vi "Find and trigger default events.vi"(9 "Event to Trigger":string, 10 "Module Lib":refnum<vi>, 11 "References Map":map{string, refnum<vi>}(c390)) -> (0 "error out":errorcluster)   [LabVIEW 2020, in "Panter Dashboard.lvlib"]
uses:
  Panter Dashboard.lvlib
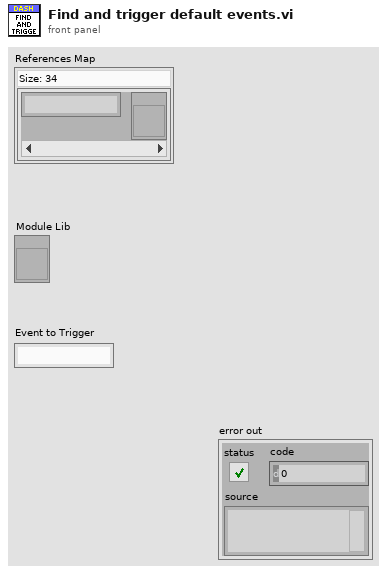
[diagram p1: front panel]
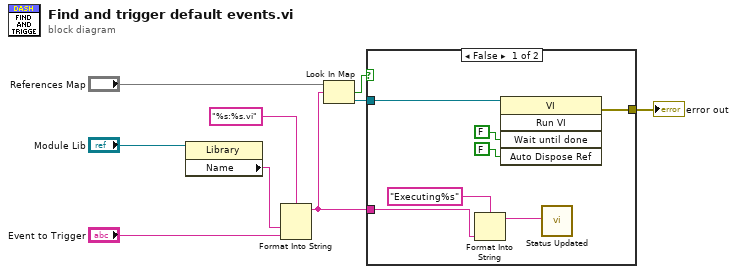
[diagram p0: block diagram]
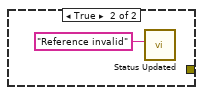
[diagram p2: hidden frame]
diagram:
  n1 = property class="Library"(reference="Module Lib") -> ("Name"=w3:string)  [unwired: 1 in, 2 out]
  n2 = Format Into String(format string="%s:%s.vi", w3, "Event to Trigger") -> (resulting string=w1:string)  [unwired: 2 in, 1 out]
  n3 = Look In Map(map="References Map", key=w1) -> (key not found?=w2:bool, value=w8:refnum<vi>)  [unwired: 1 in]
  n4 = case shown="False" w2 {
    tunnel: w8 -> [w13 _]
    tunnel: [w16 _] -> w9
    tunnel: w1 -> [w11 _]
    frame False {
      n5 = Format Into String(format string="Executing%s" ("Status"), w11) -> (resulting string=w10:string)  [unwired: 2 in, 1 out]
      n6 = invoke class="VI" method="Run VI"(reference=w13, "Wait until done"=FALSE ("Wait Until Done"), "Auto Dispose Ref"=FALSE ("Auto Dispose Reference")) -> (error out=w16:errorcluster)  [unwired: 2 in, 4 out]
      n7 = call "Status Updated.vi"("Status"=w10) -> ()  [unwired: 10 in, 1 out]
    }
    frame True {
      n8 = call "Status Updated.vi"("Status"="Reference invalid") -> ()  [unwired: 10 in, 1 out]
    }
  }
  "error out" <- w9
